vi "cluster_save.vi"(10 "INI Fomatted Cluster":variant, 11 "FileSavePath":path=path "d:/bb.ini") -> (3 "FilePath":path=path "d:/bb.ini")   [LabVIEW 2011]
uses:
  <vilib>/Utility/config.llb/NI_LVConfig.lvlib
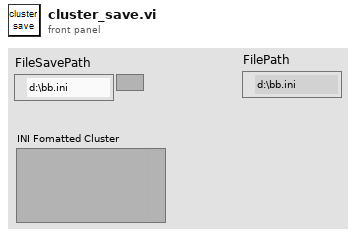
[diagram p1: front panel]
types:
  T1 = typedef "NI_LVConfig.lvlib/Config Data RefNum.ctl" = refnum<k1>
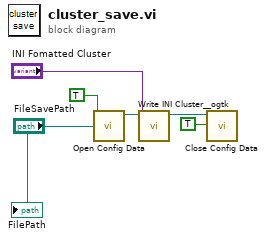
[diagram p0: block diagram]
diagram:
  n1 = call <vilib>:"Open Config Data.vi"("create file if necessary (T)"=TRUE, "configuration file path"="FileSavePath") -> ("refnum"=w6:T1)  [unwired: 7 in, 2 out]
  n2 = call <userlib>:"Write INI Cluster__ogtk.vi"("INI Fomatted Cluster"="INI Fomatted Cluster", "refnum"=w6) -> ("dup refnum"=w4:T1)  [unwired: 8 in, 1 out]
  n3 = call <vilib>:"Close Config Data.vi"("write file if changed (T)"=TRUE, "refnum"=w4) -> ()  [unwired: 8 in, 2 out]
  "FilePath" <- "FileSavePath"
